vi "DuALEX_NG.vi"() -> ()   [LabVIEW 2011]
uses:
  <vilib>/DAQmx/write.llb/DAQmx Write (Analog Wfm 1Chan NSamp).vi
  <vilib>/DAQmx/create/channels.llb/DAQmx Create Channel (AO-Voltage-Basic).vi
  <vilib>/DAQmx/configure/timing.llb/DAQmx Timing (Sample Clock).vi
  <vilib>/DAQmx/create/channels.llb/DAQmx Create Channel (CO-Pulse Generation-Frequency).vi
  <vilib>/DAQmx/configure/events/hardwareSignals.llb/DAQmx Export Signal (Most Signals).vi
  <vilib>/DAQmx/configure/trigger.llb/DAQmx Start Trigger (Digital Edge).vi
  <vilib>/DAQmx/configure/timing.llb/DAQmx Timing (Implicit).vi
  <vilib>/DAQmx/miscellaneous.llb/DAQmx Fill In Error Info.vi
  <vilib>/measure/NI_MABase.lvlib
panel:
  in  "Analog Amplitude":dbl=1.0 format="%0.2p"
  in  "Repetition Frequency":dbl=1.0 format="%.6f"
  in  "Stop Button":bool
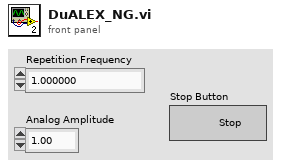
[diagram p1: front panel]
types:
  T1 = enum16{"Sine Wave", "Triangle Wave", "Square Wave", "Sawtooth Wave"}
  T2 = cluster{"Ao0 Sample Clock Rate":dbl, "Ao0 Sample Clock Rate":dbl}
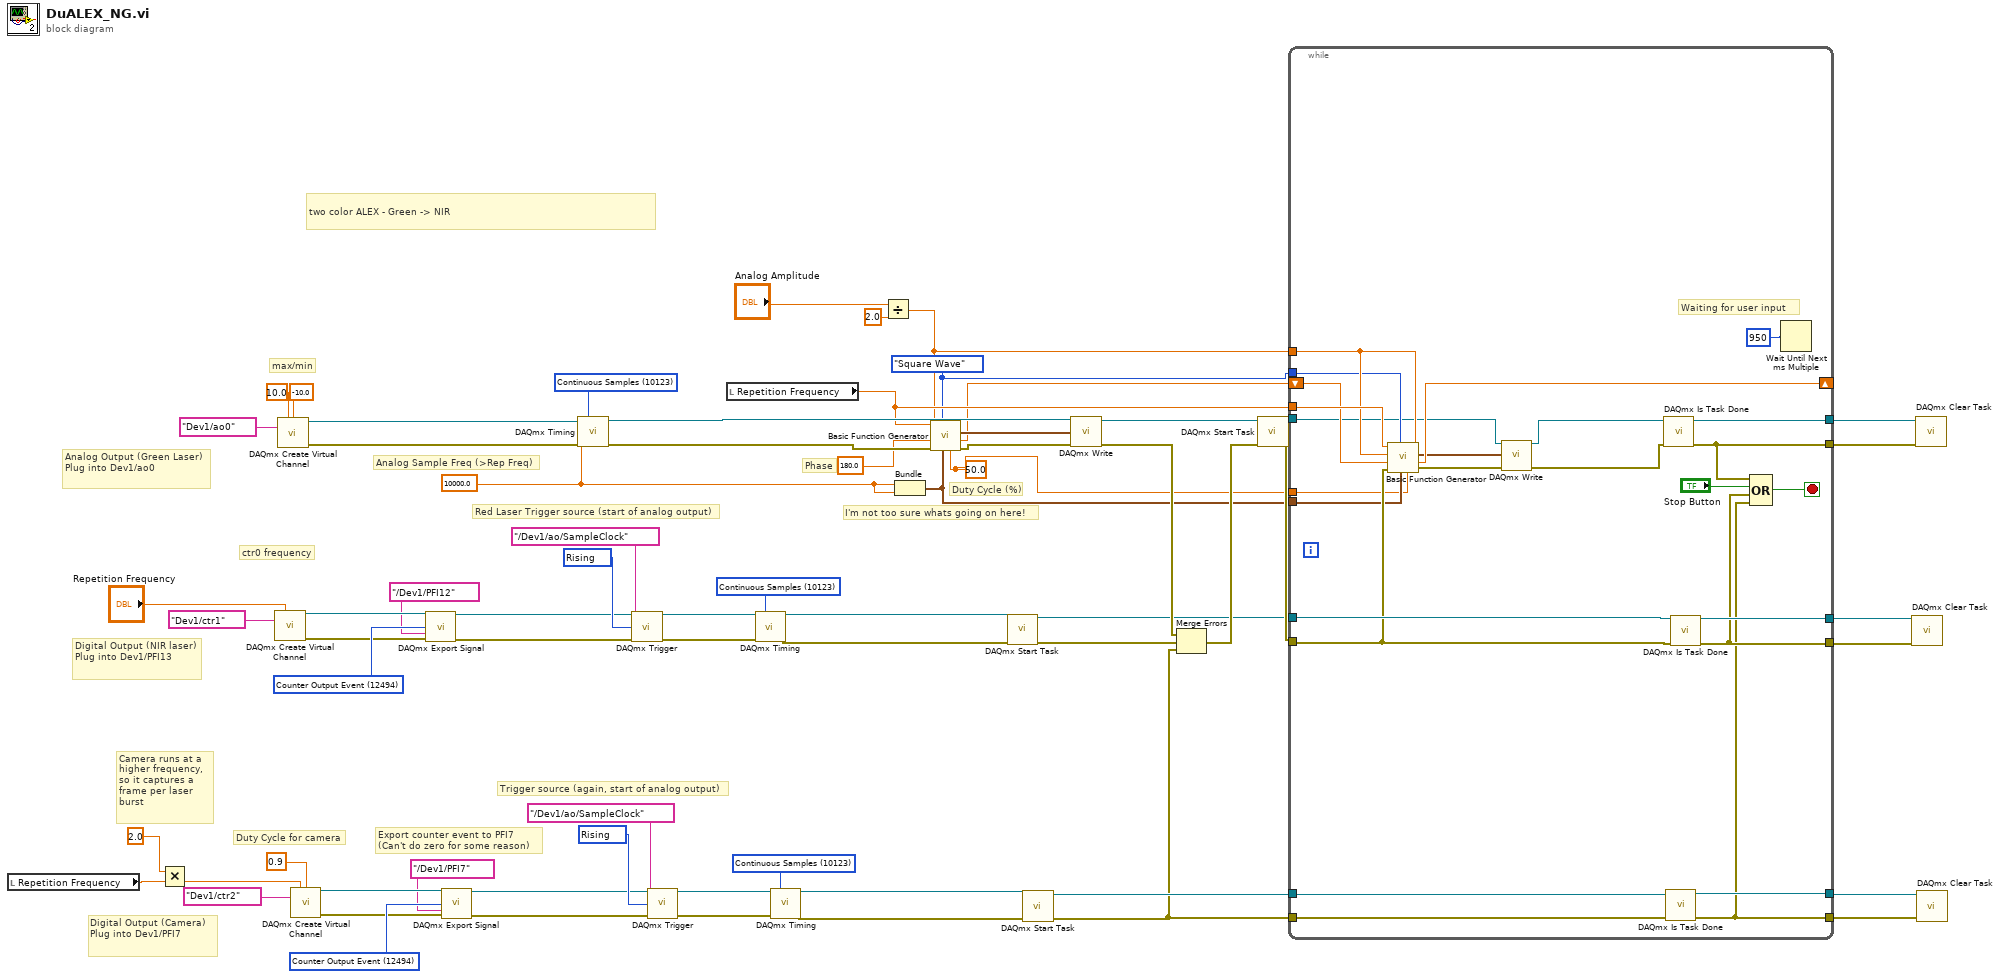
[diagram p0: block diagram]
diagram:
  w23 = 10280 items=["Rising"=10280, "Falling"=10171] ("edge")
  w26 = 10123 items=["Finite Samples"=10178, "Continuous Samples"=10123, "Hardware Timed Single Point"=12522] ("sample mode")
  w28 = 12494 items=["AI Convert Clock"=12484, "10MHz Reference Clock"=12536, "20MHz Timebase Clock"=12486, "Sample Clock"=12487, "Advance Trigger"=12488, "Reference Trigger"=12490, "Start Trigger"=12491, "Advance Complete Event"=12492, "AI Hold Complete Event"=12493, "Counter Output Event"=12494, "Change Detection Event"=12511, "Watchdog Timer Expired Event"=12512] ("signal")
  w35 = 10123 items=["Finite Samples"=10178, "Continuous Samples"=10123, "Hardware Timed Single Point"=12522] ("sample mode")
  w3 = 50.0 ("square wave duty cycle (%)")
  w1 = T1."Square Wave" ("signal type")
  w55 = 10280 items=["Rising"=10280, "Falling"=10171] ("edge")
  w60 = 10123 items=["Finite Samples"=10178, "Continuous Samples"=10123, "Hardware Timed Single Point"=12522] ("sample mode")
  w62 = 12494 items=["AI Convert Clock"=12484, "10MHz Reference Clock"=12536, "20MHz Timebase Clock"=12486, "Sample Clock"=12487, "Advance Trigger"=12488, "Reference Trigger"=12490, "Start Trigger"=12491, "Advance Complete Event"=12492, "AI Hold Complete Event"=12493, "Counter Output Event"=12494, "Change Detection Event"=12511, "Watchdog Timer Expired Event"=12512] ("signal")
  w7 = 10000.0 ("Ao0 Sample Clock Rate")
  # "two color ALEX - Green -> NIR"
  # "Duty Cycle for camera"
  # "Camera runs at a higher frequency, so it captures a frame per laser burst"
  # "Digital Output (Camera) Plug into Dev1/PFI7"
  # "Trigger source (again, start of analog output)"
  # "Export counter event to PFI7\n(Can't do zero for some reason)"
  # "Digital Output (NIR laser) Plug into Dev1/PFI13"
  # "Analog Output (Green Laser) Plug into Dev1/ao0"
  # "Duty Cycle (%)"
  # "Phase"
  # "Analog Sample Freq (>Rep Freq)"
  # "I'm not too sure whats going on here!"
  # "Red Laser Trigger source (start of analog output)"
  # "ctr0 frequency"
  # "max/min"
  n1 = local read "Repetition Frequency"() -> (w15:dbl)
  n2 = Multiply(x=2.0 ("Repetition Frequency"), y=w15) -> (x*y=w14:dbl)
  n3 = call-poly <vilib>:"DAQmx Create Virtual Channel.vi"("frequency"="Repetition Frequency", "counter"=tag "Dev1/ctr1") -> ("task out"=w63:refnum<k21>, "error out"=w61:errorcluster)  [unwired: 12 in]
  n4 = call-poly <vilib>:"DAQmx Create Virtual Channel.vi"("maximum value"=10.0, "minimum value"=-10.0, "physical channels"=tag "Dev1/ao0") -> ("task out"=w67:refnum<k21>, "error out"=w66:errorcluster)  [unwired: 11 in]
  n5 = call-poly <vilib>:"DAQmx Create Virtual Channel.vi"("frequency"=w14, "duty cycle"=0.9, "counter"=tag "Dev1/ctr2") -> ("task out"=w29:refnum<k21>, "error out"=w27:errorcluster)  [unwired: 11 in]
  n6 = call-poly <vilib>:"DAQmx Export Signal.vi"("task/channels in"=w63, "signal"=w62, "output terminal"=tag "/Dev1/PFI12", "error in"=w61) -> ("task out"=w54:refnum<k21>, "error out"=w51:errorcluster)  [unwired: 10 in]
  n7 = call-poly <vilib>:"DAQmx Export Signal.vi"("task/channels in"=w29, "signal"=w28, "output terminal"=tag "/Dev1/PFI7", "error in"=w27) -> ("task out"=w22:refnum<k21>, "error out"=w19:errorcluster)  [unwired: 10 in]
  n8 = call-poly <vilib>:"DAQmx Timing.vi"("task/channels in"=w67, "sample mode"=w35, "rate"=w7, "error in"=w66) -> ("task out"=w59:refnum<k21>, "error out"=w58:errorcluster)  [unwired: 10 in]
  n9 = call-poly <vilib>:"DAQmx Trigger.vi"("task/channels in"=w54, "source"=tag "/Dev1/ao/SampleClock", "edge"=w55, "error in"=w51) -> ("task out"=w53:refnum<k21>, "error out"=w52:errorcluster)  [unwired: 10 in]
  n10 = call-poly <vilib>:"DAQmx Trigger.vi"("task/channels in"=w22, "source"=tag "/Dev1/ao/SampleClock", "edge"=w23, "error in"=w19) -> ("task out"=w21:refnum<k21>, "error out"=w20:errorcluster)  [unwired: 10 in]
  n11 = local read "Repetition Frequency"() -> (w6:dbl)
  n12 = call-poly <vilib>:"DAQmx Timing.vi"("task/channels in"=w53, "sample mode"=w60, "error in"=w52) -> ("task out"=w48:refnum<k21>, "error out"=w47:errorcluster)  [unwired: 11 in]
  n13 = call-poly <vilib>:"DAQmx Timing.vi"("task/channels in"=w21, "sample mode"=w26, "error in"=w20) -> ("task out"=w18:refnum<k21>, "error out"=w17:errorcluster)  [unwired: 11 in]
  n14 = Divide(x="Analog Amplitude", y=2.0) -> (x/y=w5:dbl)
  n15 = Bundle("Ao0 Sample Clock Rate"=w7, "Ao0 Sample Clock Rate"=w7) -> (w4:T2)  [unwired: 1 in]
  n16 = call <vilib>:"Basic Function Generator.vi"("offset"=w5, "square wave duty cycle (%)"=w3, "sampling info"=w4, "signal type"=w1, "error in (no error)"=w58, "phase"=180.0, "amplitude"=w5, "frequency"=w6) -> ("error out"=w49:errorcluster, "phase out"=w2:dbl, "signal out"=w50:waveform(dbl))  [unwired: 1 in]
  n17 = call <vilib>:"DAQmx Start Task.vi"("task/channels in"=w48, "error in"=w47) -> ("task out"=w36:refnum<k21>, "error out"=w46:errorcluster)  [unwired: 12 in]
  n18 = call <vilib>:"DAQmx Start Task.vi"("task/channels in"=w18, "error in"=w17) -> ("task out"=w11:refnum<k21>, "error out"=w10:errorcluster)  [unwired: 12 in]
  n19 = call-poly <vilib>:"DAQmx Write.vi"("task/channels in"=w59, "data"=w50, "error in"=w49) -> ("task out"=w43:refnum<k21>, "error out"=w45:errorcluster)  [unwired: 10 in, 1 out]
  n20 = Merge Errors(w45, w46, w10) -> (w44:errorcluster)
  n21 = call <vilib>:"DAQmx Start Task.vi"("task/channels in"=w43, "error in"=w44) -> ("task out"=w42:refnum<k21>, "error out"=w41:errorcluster)  [unwired: 12 in]
  n22 = while {
    tunnel: [w93] -> w37
    tunnel: [w86] -> w40
    tunnel: [w90] -> w38
    tunnel: [w84] -> w39
    tunnel: w42 -> [w69]
    tunnel: w41 -> [w78]
    tunnel: w36 -> [w89]
    tunnel: w11 -> [w88]
    tunnel: w10 -> [w87]
    tunnel: [w83] -> w9
    tunnel: [w82] -> w8
    tunnel: w6 -> [w77]
    tunnel: w5 -> [w76]
    tunnel: w4 -> [w75]
    tunnel: w3 -> [w74]
    shift-right: [w73] -> _
    shift-left: w2 -> [w72]
    tunnel: w1 -> [w71]
    stop <- w91 stop-if-true
    # "Waiting for user input"
    n23 = call <vilib>:"Basic Function Generator.vi"("offset"=w76, "square wave duty cycle (%)"=w74, "sampling info"=w75, "signal type"=w71, "error in (no error)"=w78, "phase"=w72, "amplitude"=w76, "frequency"=w77) -> ("error out"=w79:errorcluster, "phase out"=w73:dbl, "signal out"=w70:waveform(dbl))  [unwired: 1 in]
    n24 = call-poly <vilib>:"DAQmx Write.vi"("task/channels in"=w69, "data"=w70, "error in"=w79) -> ("task out"=w81:refnum<k21>, "error out"=w80:errorcluster)  [unwired: 10 in, 1 out]
    n25 = call <vilib>:"DAQmx Is Task Done.vi"("task/channels in"=w81, "error in"=w80) -> ("task out"=w93:refnum<k21>, "error out"=w86:errorcluster)  [unwired: 11 in, 1 out]
    n26 = call <vilib>:"DAQmx Is Task Done.vi"("task/channels in"=w88, "error in"=w87) -> ("task out"=w83:refnum<k21>, "error out"=w82:errorcluster)  [unwired: 11 in, 1 out]
    n27 = call <vilib>:"DAQmx Is Task Done.vi"("task/channels in"=w89, "error in"=w78) -> ("task out"=w90:refnum<k21>, "error out"=w84:errorcluster)  [unwired: 11 in, 1 out]
    n28 = Compound Arithmetic op=OR(w86, "Stop Button", w84, w82) -> (w91:bool)
    n29 = Wait Until Next ms Multiple(millisecond multiple=u32 950) -> ()  [unwired: 1 out]
  }
  n30 = call <vilib>:"DAQmx Clear Task.vi"("task in"=w38, "error in"=w39) -> ()  [unwired: 13 in, 1 out]
  n31 = call <vilib>:"DAQmx Clear Task.vi"("task in"=w37, "error in"=w40) -> ()  [unwired: 13 in, 1 out]
  n32 = call <vilib>:"DAQmx Clear Task.vi"("task in"=w9, "error in"=w8) -> ()  [unwired: 13 in, 1 out]
